vi "Tokenize JSON.vi"(8 "error in":errorcluster, 11 "JSON String":string="{\n   \"data\":[\n      {\n         \"message\":{\n            \"content\":{\n               \"type\":\"text/plain\",\n               \"text\":\"Some text asd\"\n            },\n            \"subject\":\"My subject\",\n            \"status\":\"published\",\n            \"replyCount\":4.8,\n            \"likeCount\":0.7\n         }\n      }\n   ]\n}") -> (0 "error out":errorcluster, 2 "Variable Names":string[](array[string]), 3 "Token Array":T1[](array[typedef]))   [LabVIEW 2015]
uses:
  Type Definitions/JSON token.ctl
  <vilib>/regexp/Match Regular Expression.xnode
panel:
  out "whole match":string
  out "Array":string[](array[string])
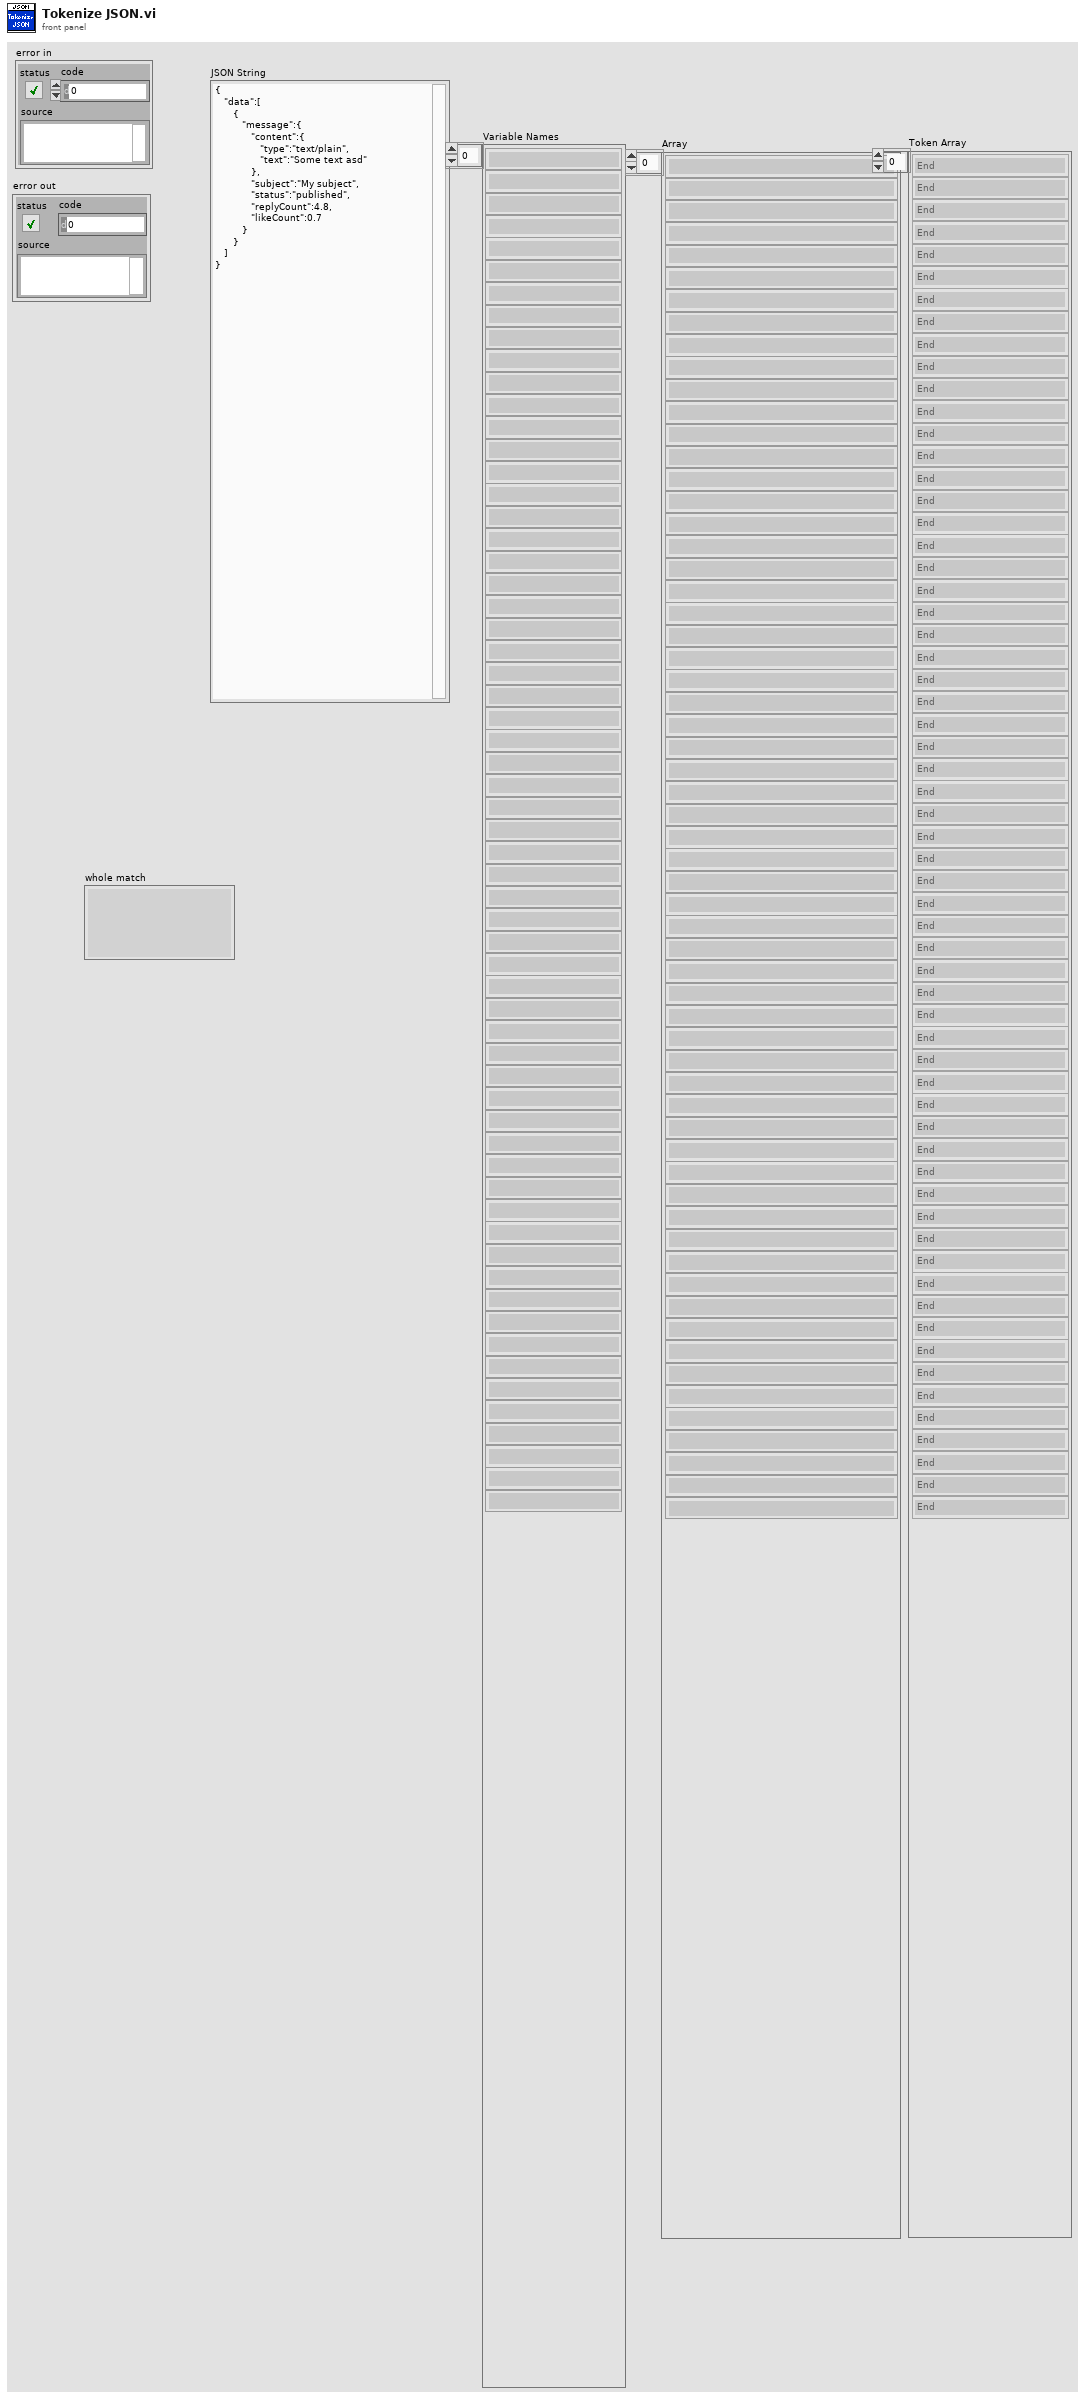
[diagram p1: front panel]
types:
  T1 = typedef "JSON token.ctl" = enum16{"I32", "New Row (2D Array)", "Decimal", "End", "Boolean", "Named Cluster", "Unnamed Cluster", "Array", "String", "FloatingPoint", "End Array", "Object of Arrays", "End Cluster", "Date and Time Stamp", "enum", "End 2D Array", "2D Array"}
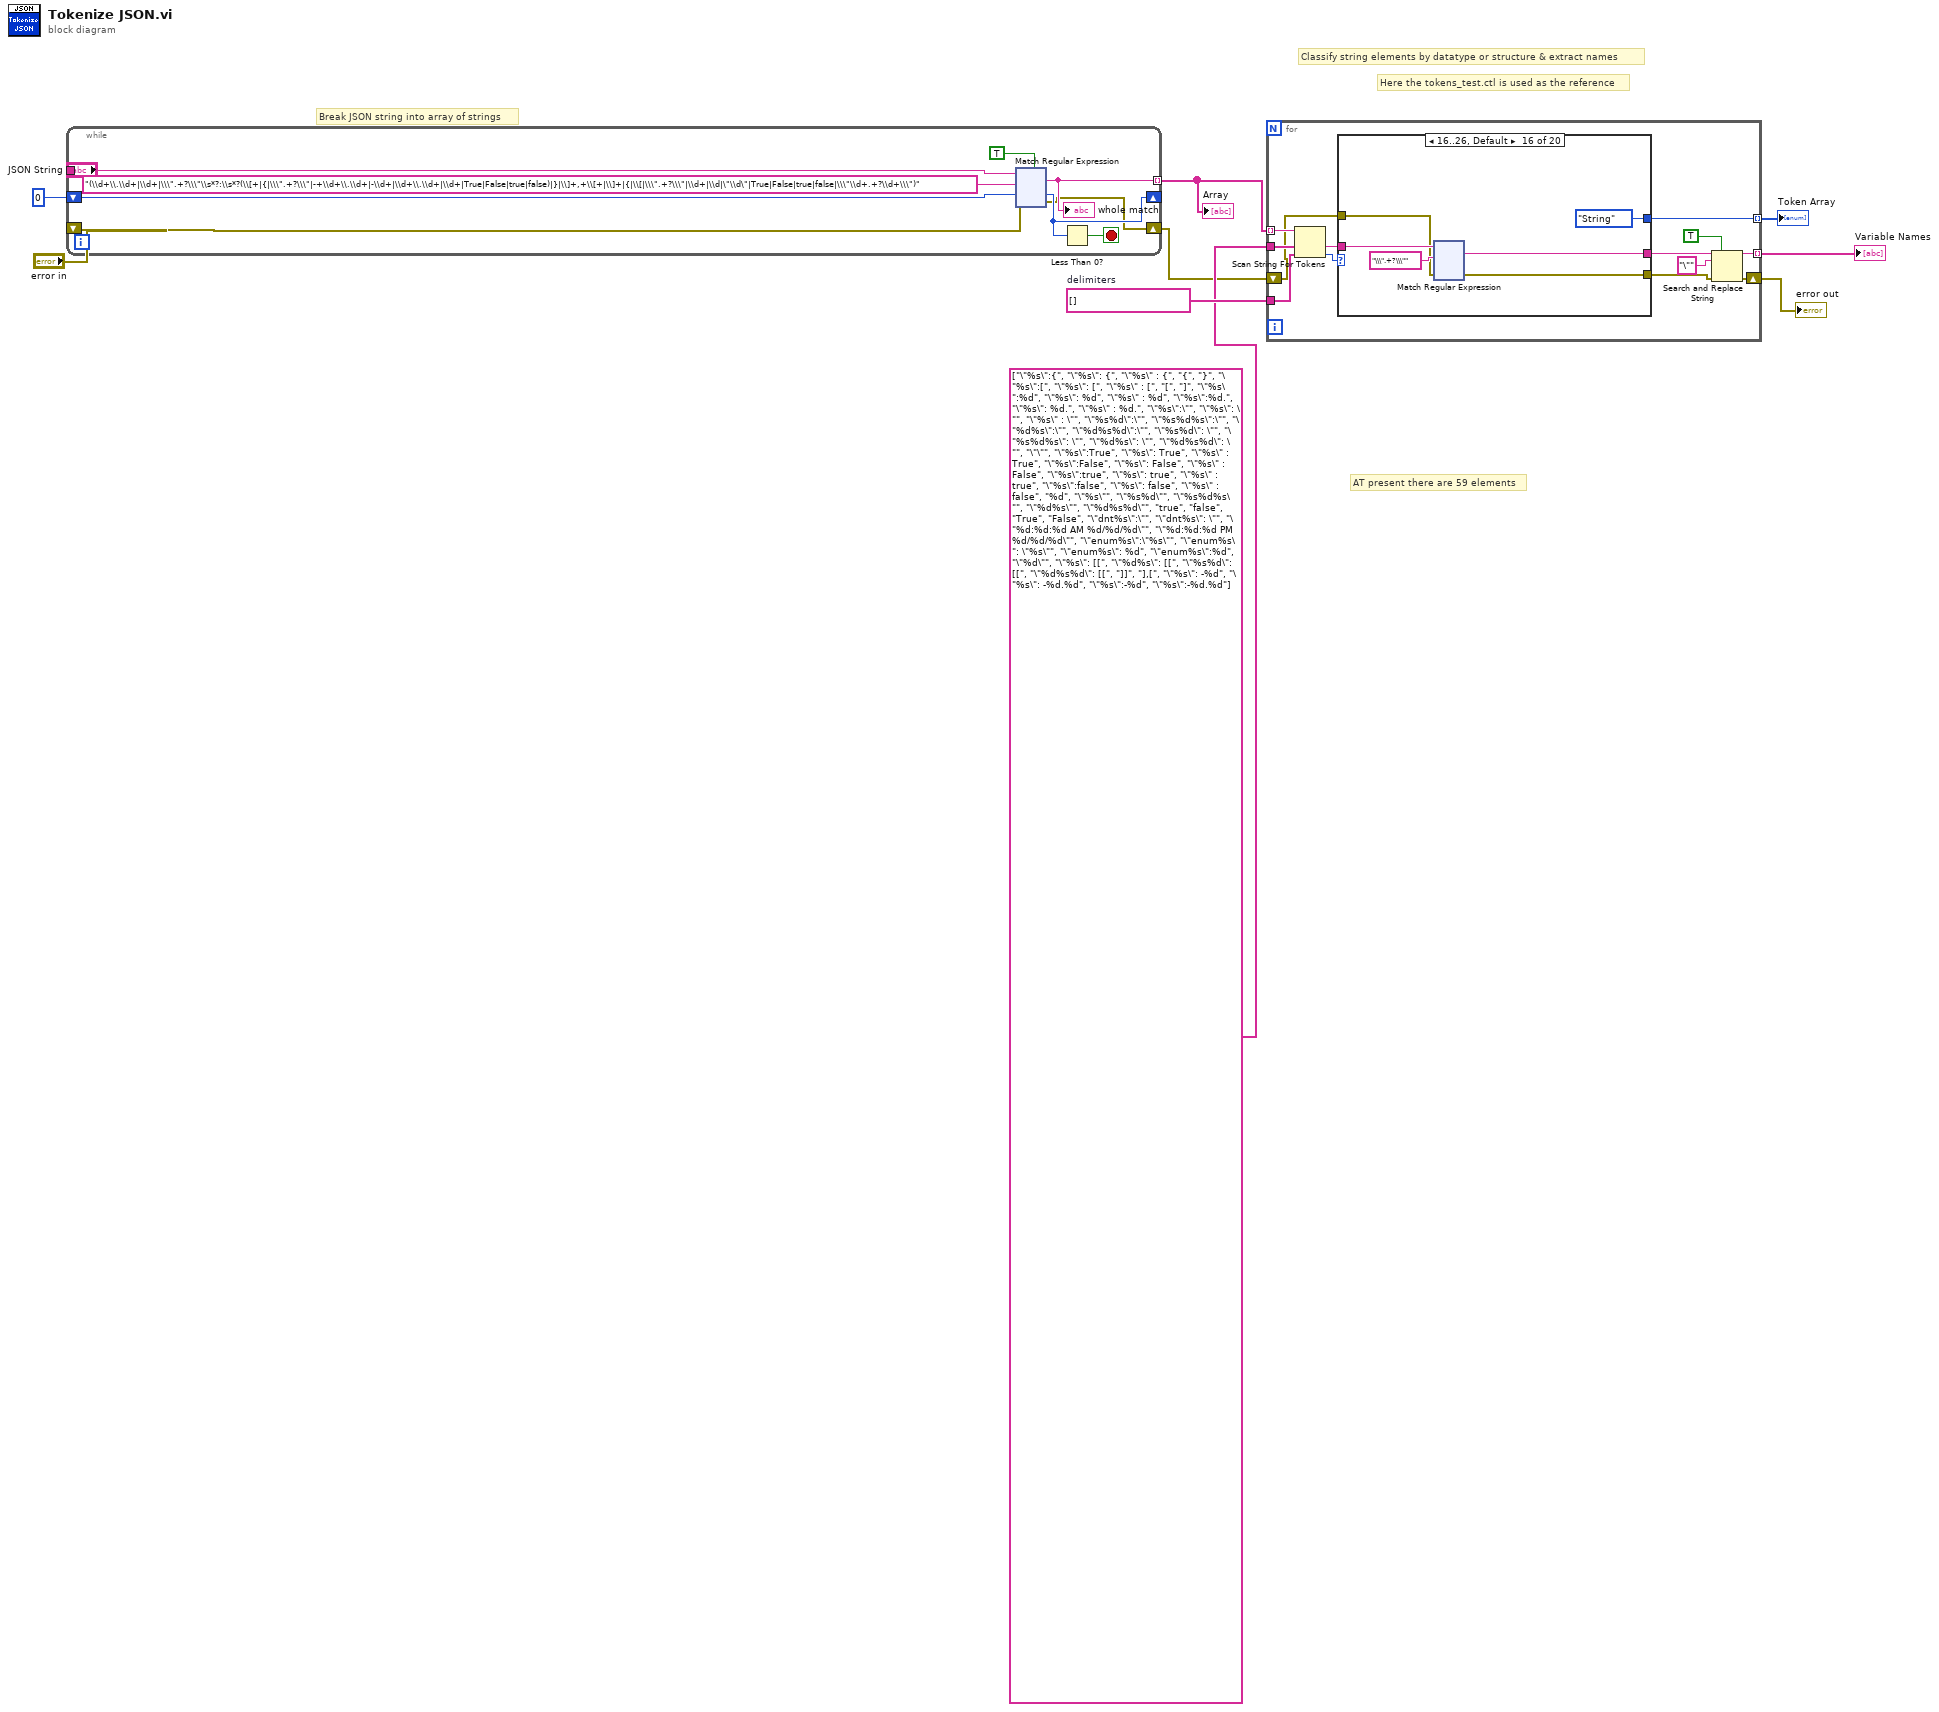
[diagram p0: block diagram]
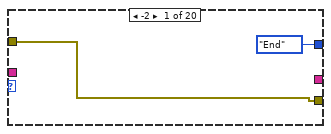
[diagram p2: hidden frame]
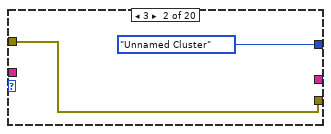
[diagram p3: hidden frame]
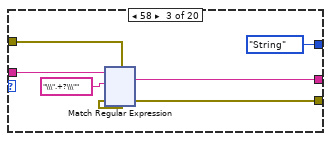
[diagram p4: hidden frame]
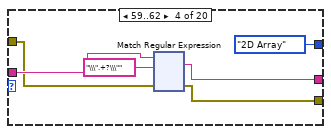
[diagram p5: hidden frame]
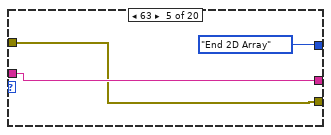
[diagram p6: hidden frame]
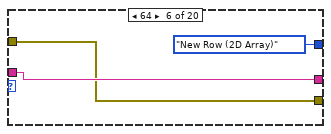
[diagram p7: hidden frame]
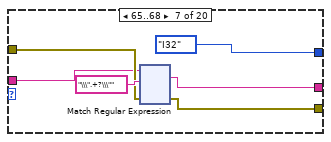
[diagram p8: hidden frame]
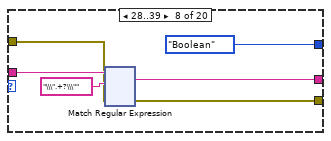
[diagram p9: hidden frame]
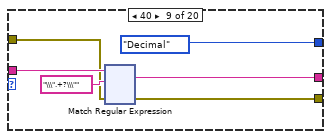
[diagram p10: hidden frame]
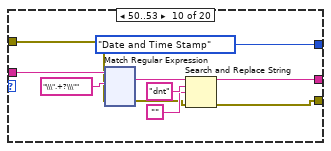
[diagram p11: hidden frame]
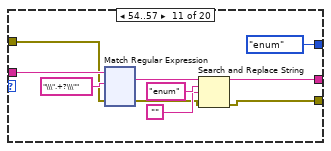
[diagram p12: hidden frame]
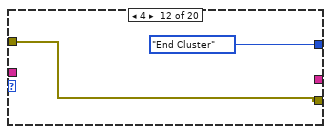
[diagram p13: hidden frame]
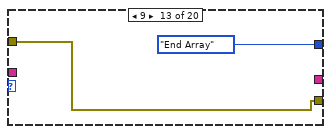
[diagram p14: hidden frame]
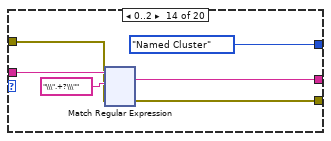
[diagram p15: hidden frame]
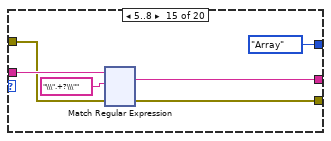
[diagram p16: hidden frame]
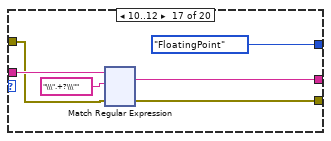
[diagram p17: hidden frame]
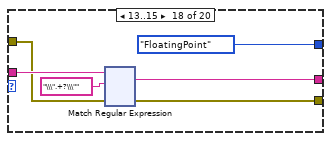
[diagram p18: hidden frame]
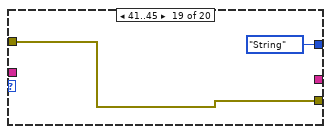
[diagram p19: hidden frame]
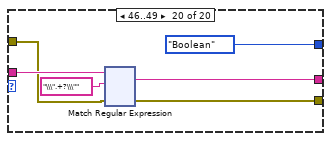
[diagram p20: hidden frame]
diagram:
  w8 = string[] []  # delimiters
  # "AT present there are 59 elements"
  # "Here the tokens_test.ctl is used as the reference"
  # "Classify string elements by datatype or structure & extract names"
  # "Break JSON string into array of strings"
  n1 = while {
    tunnel: "JSON String" -> [w18]
    shift-right: [w13] -> _
    shift-left: 0 ("offset past match") -> [w16]
    tunnel: [w15] -> w7 mode=indexing
    shift-right: [w11] -> w3
    shift-left: "error in" -> [w12]
    stop <- w19 stop-if-true
    n2 = xnode "Match Regular Expression"("input string"=w18, "regular expression"="(\\d+\\.\\d+|\\d+|\\\".+?\\\"\\s*?:\\s*?(\\[+|{|\\\".+?\\\"|-+\\d+\\.\\d+|-\\d+|\\d+\\.\\d+|\\d+|True|False|true|false)|}|\\]+,+\\[+|\\]+|{|\\[|\\\".+?\\\"|\\d+|\\d|\"\\d\"|True|False|true|false|\\\"\\d+.+?\\d+\\\")", "offset (0)"=w16, "error in"=w12, "multiline? (F)"=TRUE) -> ("whole match"=w15:string, "offset past match"=w13:i32, "error out"=w11:errorcluster)  [unwired: 1 in, 2 out]
    "whole match" <- w15
    n3 = Less Than 0?(x=w13) -> (x < 0?=w19:bool)
  }
  "Array" <- w7
  n4 = for {
    tunnel: w7 -> [w137] mode=indexing
    tunnel: w8 -> [w146]
    tunnel: string[] ["\"%s\":{", "\"%s\": {", "\"%s\" : {", "{", "}", "\"%s\":[", "\"%s\": [", "\"%s\" : [", "[", "]", "\"%s\":%d", "\"%s\": %d", "\"%s\" : %d", "\"%s\":%d.", "\"%s\": %d.", "\"%s\" : %d.", "\"%s\":\"", "\"%s\": \"", "\"%s\" : \"", "\"%s%d\":\"", "\"%s%d%s\":\"", "\"%d%s\":\"", "\"%d%s%d\":\"", "\"%s%d\": \"", "\"%s%d%s\": \"", "\"%d%s\": \"", "\"%d%s%d\": \"", "\"\"", "\"%s\":True", "\"%s\": True", "\"%s\" : True", "\"%s\":False", "\"%s\": False", "\"%s\" : False", "\"%s\":true", "\"%s\": true", "\"%s\" : true", "\"%s\":false", "\"%s\": false", "\"%s\" : false", "%d", "\"%s\"", "\"%s%d\"", "\"%s%d%s\"", "\"%d%s\"", "\"%d%s%d\"", "true", "false", "True", "False", "\"dnt%s\":\"", "\"dnt%s\": \"", "\"%d:%d:%d AM %d/%d/%d\"", "\"%d:%d:%d PM %d/%d/%d\"", "\"enum%s\":\"%s\"", "\"enum%s\": \"%s\"", "\"enum%s\": %d", "\"enum%s\":%d", "\"%d\"", "\"%s\": [[", "\"%d%s\": [[", "\"%s%d\": [[", "\"%d%s%d\": [[", "]]", "],[", "\"%s\": -%d", "\"%s\": -%d.%d", "\"%s\":-%d", "\"%s\":-%d.%d"] ("Array 2") -> [w145]
    tunnel: [w144] -> w5 mode=indexing
    tunnel: [w141] -> w6 mode=indexing
    shift-right: [w134] -> w2
    shift-left: w3 -> [w136]
    n5 = Scan String For Tokens(6:w146, 7:w145, 9:w137) -> (0:w138:i32, 1:w143:string)  [unwired: 3 in, 2 out]
    n6 = case shown="16..26, Default" w138 {
      tunnel: [JSON_token."End" JSON_token."Unnamed Cluster" JSON_token."String" JSON_token."2D Array" JSON_token."End 2D Array" JSON_token."New Row (2D Array)" JSON_token."I32" JSON_token."Boolean" JSON_token."Decimal" JSON_token."Date and Time Stamp" JSON_token."enum" JSON_token."End Cluster" JSON_token."End Array" JSON_token."Named Cluster" JSON_token."Array" JSON_token."String" JSON_token."FloatingPoint" JSON_token."FloatingPoint" JSON_token."String" JSON_token."Boolean"] -> w144
      tunnel: w143 -> [_ _ w155 w275 w392 w396 w398 w519 w641 w764 w888 _ _ w1012 w1132 w1252 w1372 w1492 _ w1614]
      tunnel: [_ _ w154 w271 w392 w396 w397 w520 w640 w760 w884 _ _ w1011 w1131 w1251 w1371 w1491 _ w1613] -> w142
      tunnel: w136 -> [w147 w149 w152 w274 w391 w394 w400 w518 w639 w759 w883 w1005 w1007 w1010 w1130 w1250 w1370 w1490 w1609 w1612]
      tunnel: [w147 w149 w151 w273 w391 w394 w399 w517 w638 w757 w881 w1005 w1007 w1009 w1129 w1249 w1369 w1489 w1609 w1611] -> w135
      frame -2 {
      }
      frame 3 {
      }
      frame 58 {
        n7 = xnode "Match Regular Expression"("input string"=w155, "regular expression"="\\\".+?\\\"", "error in"=w152) -> ("whole match"=w154:string, "error out"=w151:errorcluster)  [unwired: 3 in, 3 out]
      }
      frame 59..62 {
        n8 = xnode "Match Regular Expression"("input string"=w275, "regular expression"="\\\".+?\\\"", "error in"=w274) -> ("whole match"=w271:string, "error out"=w273:errorcluster)  [unwired: 3 in, 3 out]
      }
      frame 63 {
      }
      frame 64 {
      }
      frame 65..68 {
        n9 = xnode "Match Regular Expression"("input string"=w398, "regular expression"="\\\".+?\\\"", "error in"=w400) -> ("whole match"=w397:string, "error out"=w399:errorcluster)  [unwired: 3 in, 3 out]
      }
      frame 28..39 {
        n10 = xnode "Match Regular Expression"("input string"=w519, "regular expression"="\\\".+?\\\"", "error in"=w518) -> ("whole match"=w520:string, "error out"=w517:errorcluster)  [unwired: 3 in, 3 out]
      }
      frame 40 {
        n11 = xnode "Match Regular Expression"("input string"=w641, "regular expression"="\\\".+?\\\"", "error in"=w639) -> ("whole match"=w640:string, "error out"=w638:errorcluster)  [unwired: 3 in, 3 out]
      }
      frame 50..53 {
        n12 = xnode "Match Regular Expression"("input string"=w764, "regular expression"="\\\".+?\\\"", "error in"=w759) -> ("whole match"=w761:string, "error out"=w758:errorcluster)  [unwired: 3 in, 3 out]
        n13 = Search and Replace String(input string=w761, search string="dnt", replace string="", error in=w758) -> (result string=w760:string, error out=w757:errorcluster)  [unwired: 4 in, 2 out]
      }
      frame 54..57 {
        n14 = xnode "Match Regular Expression"("input string"=w888, "regular expression"="\\\".+?\\\"", "error in"=w883) -> ("whole match"=w887:string, "error out"=w882:errorcluster)  [unwired: 3 in, 3 out]
        n15 = Search and Replace String(input string=w887, search string="enum", replace string="", error in=w882) -> (result string=w884:string, error out=w881:errorcluster)  [unwired: 4 in, 2 out]
      }
      frame 4 {
      }
      frame 9 {
      }
      frame 0..2 {
        n16 = xnode "Match Regular Expression"("input string"=w1012, "regular expression"="\\\".+?\\\"", "error in"=w1010) -> ("whole match"=w1011:string, "error out"=w1009:errorcluster)  [unwired: 3 in, 3 out]
      }
      frame 5..8 {
        n17 = xnode "Match Regular Expression"("input string"=w1132, "regular expression"="\\\".+?\\\"", "error in"=w1130) -> ("whole match"=w1131:string, "error out"=w1129:errorcluster)  [unwired: 3 in, 3 out]
      }
      frame 16..26, Default {
        n18 = xnode "Match Regular Expression"("input string"=w1252, "regular expression"="\\\".+?\\\"", "error in"=w1250) -> ("whole match"=w1251:string, "error out"=w1249:errorcluster)  [unwired: 3 in, 3 out]
      }
      frame 10..12 {
        n19 = xnode "Match Regular Expression"("input string"=w1372, "regular expression"="\\\".+?\\\"", "error in"=w1370) -> ("whole match"=w1371:string, "error out"=w1369:errorcluster)  [unwired: 3 in, 3 out]
      }
      frame 13..15 {
        n20 = xnode "Match Regular Expression"("input string"=w1492, "regular expression"="\\\".+?\\\"", "error in"=w1490) -> ("whole match"=w1491:string, "error out"=w1489:errorcluster)  [unwired: 3 in, 3 out]
      }
      frame 41..45 {
      }
      frame 46..49 {
        n21 = xnode "Match Regular Expression"("input string"=w1614, "regular expression"="\\\".+?\\\"", "error in"=w1612) -> ("whole match"=w1613:string, "error out"=w1611:errorcluster)  [unwired: 3 in, 3 out]
      }
    }
    n22 = Search and Replace String(replace all?=TRUE ("replace all? (F)"), input string=w142, search string="\"", error in=w135) -> (result string=w141:string, error out=w134:errorcluster)  [unwired: 4 in, 2 out]
  }
  "Variable Names" <- w6
  "Token Array" <- w5
  "error out" <- w2
